vi "Punto 6.vi"() -> ()   [LabVIEW 2020]
panel:
  out "number of replacements":i32
  in  "Boolean":bool
  in  "String":string
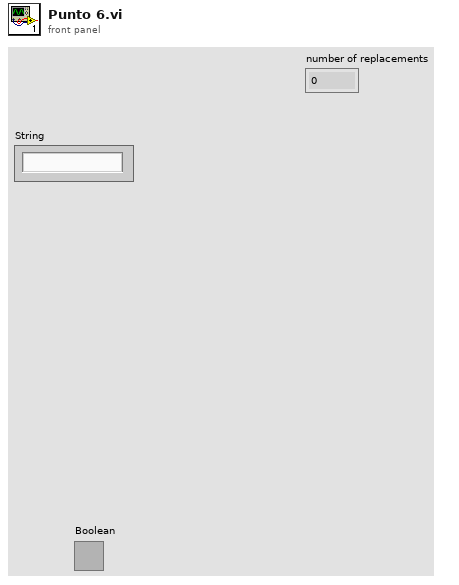
[diagram p1: front panel]
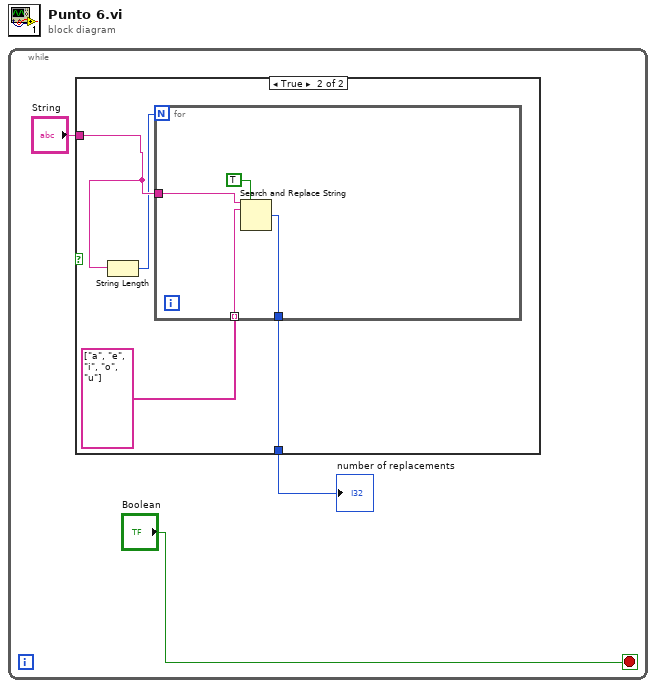
[diagram p0: block diagram]
diagram:
  n1 = while {
    stop <- "Boolean" stop-if-true
    n2 = case shown="True" {
      selector: _ -> [_ _]
      tunnel: "String" -> [_ w7]
      tunnel: [_ w4] -> w1
      frame False {
      }
      frame True {
        n3 = String Length(string=w7) -> (length=w5:i32)
        n4 = for {
          N: w5 -> [_]
          tunnel: w7 -> [w10]
          tunnel: string[] ["a", "e", "i", "o", "u"] -> [w9] mode=indexing
          tunnel: [w8] -> w4
          n5 = Search and Replace String(replace all?=TRUE, input string=w10, search string=w9) -> (number of replacements=w8:i32)  [unwired: 5 in, 3 out]
        }
      }
    }
    "number of replacements" <- w1
  }
